vi "merge_Edge Detect.vi"   [LabVIEW 2017, in "NI_FunctionBlockMergeVIs.lvlib"]
doc: "Detects rising edges on <B>input 1</B> and falling edges on <B>input 2</B>. The <B>output</B> indicator pulses TRUE for one iteration when <B>input 1</B> transitions to TRUE, when <B>input 2</B> transitions to FALSE, or when both conditions occur simultaneously."
uses:
  <vilib>/functionblocks/NI_FunctionBlockMergeVIs.lvlib
  <vilib>/functionblocks/FB Core/FB Core.xnode
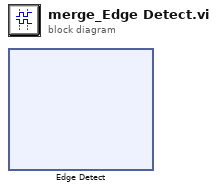
[diagram p0: block diagram]
diagram:
  n1 = xnode "Edge Detect"() -> ()  [unwired: 3 in, 2 out]
